vi "UDP rd_lbne.vi"(1 "ADDRESS 2":i16) -> (0 "DATA 2":u32 format="%x")   [LabVIEW 2014]
doc: "This VI is designed to be used with the UDP Receiver VI. Run the UDP Receiver.vi first.\n\nThe UDP protocol differs from TCP in that there is no error-checking with the packets of information that are sent, and thus no guarantee whatsoever that an intended recipient will actually receive a given piece of data.\n\nUDP does offer the ability to \"broadcast\" data across a network--simply specify an IP Address of all ones (255.255.255.255) to attempt to broadcast information network-wide. Keep in mind that routers and other network hardware will generally refuse to forward the broadcast beyond certain points, so the extent of the broadcast will in practice be limited."
uses:
  D:/share/LIQ_ARG/LBNE_SW/LBNE_DLL/LBNE_DLL/bin/Debug/LBNE_DLL.dll
  LBNE_DLL/LBNE_DLL/bin/Debug/LBNE_DLL.dll
  LBNE_Global .vi
panel:
  out "REG_RD":string
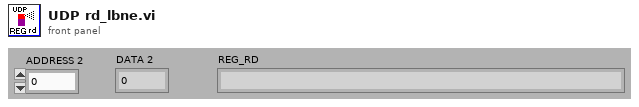
[diagram p1: front panel]
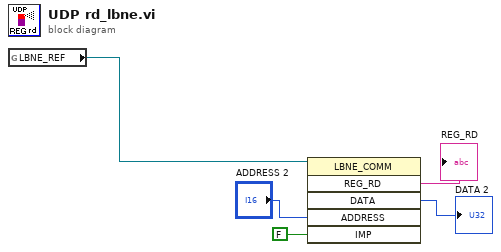
[diagram p0: block diagram]
diagram:
  n1 = global read "LBNE_Global .vi" "LBNE_REF"() -> (w1:refnum<k24>)
  n2 = invoke class="LBNE_COMM" method="REG_RD"(reference=w1, "ADDRESS"="ADDRESS 2", "IMP"=FALSE) -> ("REG_RD"=→"REG_RD":string, "DATA"=→"DATA 2":u32)  [unwired: 3 in, 4 out]
